vi "BLED1112-Rx Packet parser (EVENT-Connection status).vi"(5 "message package":u8[](array[numeric])=[128, 16, 3, 0, 0, 9, 198, 109, 145, 234, 23, 0, 0, 6, 0, 100, 0, 0, 0, 255] format="%02x") -> (0 "message out":u8[](array[numeric])=[128, 16, 3, 0, 0, 9, 198, 109, 145, 234, 23, 0, 0, 6, 0, 100, 0, 0, 0, 255] format="%02x", 1 "Packet OK":bool, 2 "Data Structure":T1={"Message Type (Response)"=128, "Payload length"=16, "Command Class (System)"=3, "Message ID"=0, "Connection handle"=0, "flags"=9, "Bluetooth address"=[198, 109, 145, 234, 23, 0], "address type"=0, "conn_interval(ms)"=7.5, "timeout(ms)"=1000.0, "latency"=0, "bonding(0xFF)"=255} {"address type" format="%02x" items=["Public", "Random"]; "flags" format="%02x"; "bonding(0xFF)" format="%02x"; "latency" format="%04x"; "Bluetooth address" format="%02x"; "Connection handle" format="%02x"; "Message ID" format="%02x"; "Message Type (Response)" format="%02x" items=["Command / Response"=0, "Event"=128]; "Command Class (System)" format="%02x" items=["System", "Persistent Store", "Attribute database", "Connection", "Attribute client", "Security Manager", "Generic Access Profile", "Hardware"]})   [LabVIEW 2015]
uses:
  Lib_Bled112 toolkit/type_def/message_type.ctl
  Lib_Bled112 toolkit/type_def/message_class.ctl
panel:
  # "Rx Packet parser (EVENT-Connection status)"
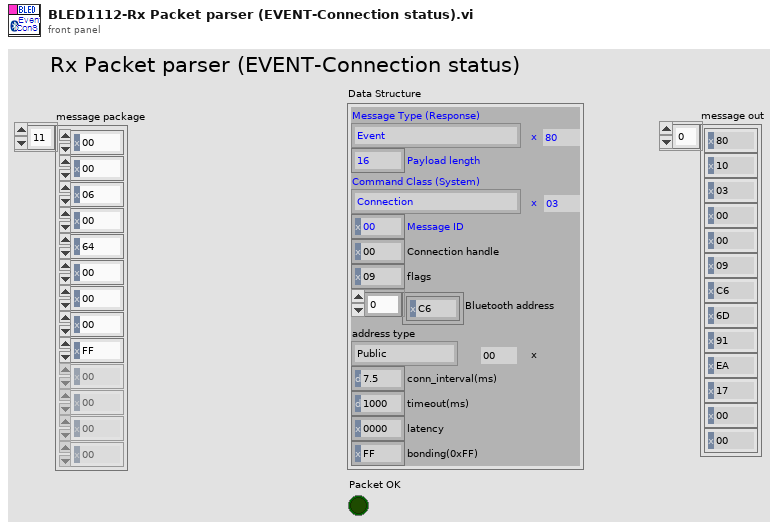
[diagram p1: front panel]
types:
  T1 = typedef "컨트롤-BLED Rx (EVENT-Connection status).ctl" = cluster{"Message Type (Response)":T2, "Payload length":u8, "Command Class (System)":T3, "Message ID":u8, "Connection handle":u8, "flags":u8, "Bluetooth address":u8[], "address type":T3, "conn_interval(ms)":dbl, "timeout(ms)":dbl, "latency":u16, "bonding(0xFF)":u8}
  T2 = typedef "message_type.ctl" = u8
  T3 = typedef "message_class.ctl" = u8
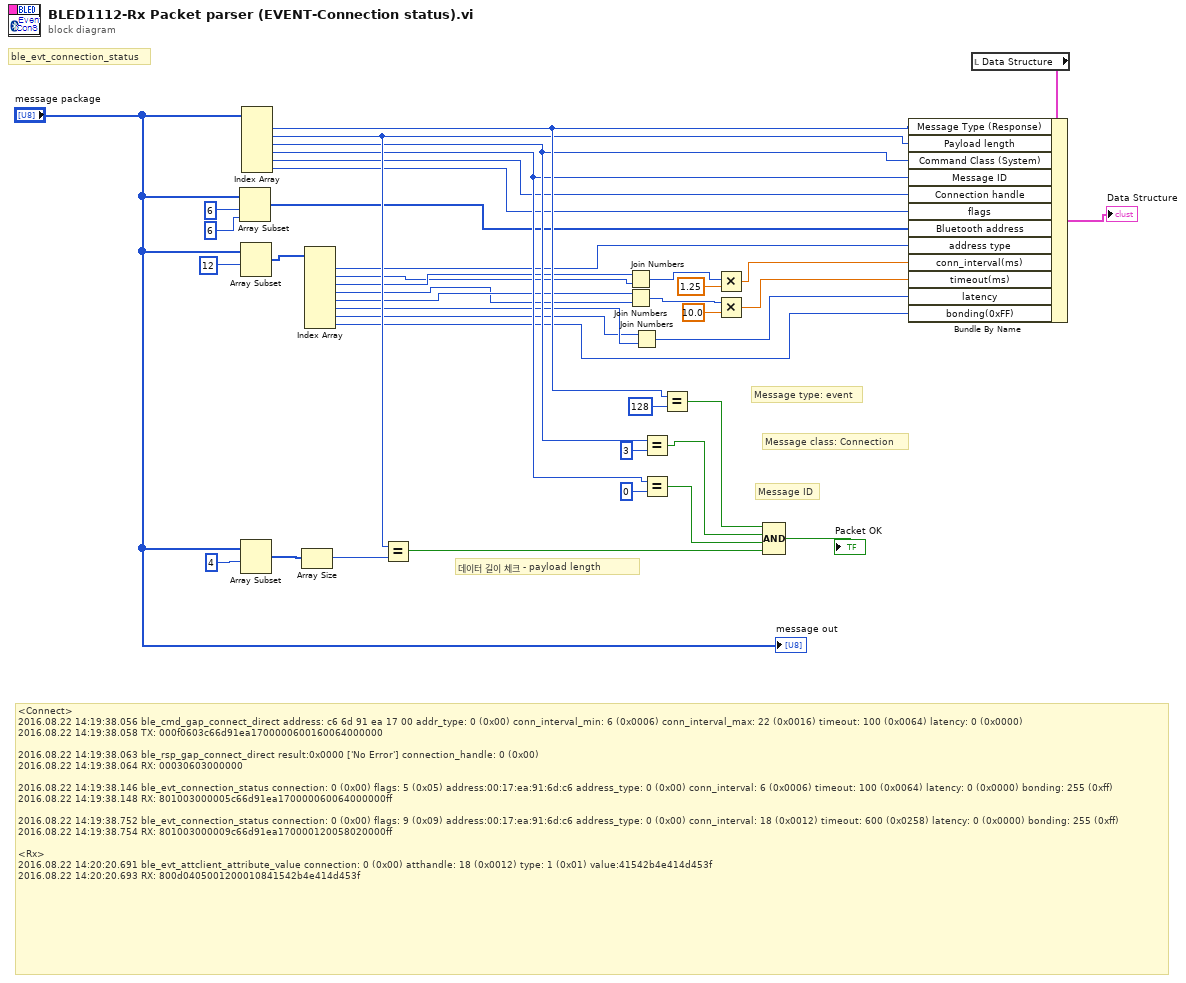
[diagram p0: block diagram]
diagram:
  # "Message type: event"
  # "ble_evt_connection_status"
  # "Message ID"
  # "Message class: Connection"
  # "데이터 길이 체크 - payload length"
  # "<Connect>\n2016.08.22 14:19:38.056 ble_cmd_gap_connect_direct address: c6 6d 91 ea 17 00 addr_type: 0 (0x00) conn_interval_min: 6 (0x0006) conn_interval_max: 22 (0x0016) timeout: 100 (0x0064) latency: 0 (0x0000)\n2016.08.22 14:19:38.058 TX: 000f0603c66d91ea1700000600160064000000\n\n2016.08.22 14:19:38.063 ble_rsp_gap_connect_direct result:0x0000 ['No Error'] connection_handle: 0 (0x00)\n2016.08.22 14:19:38.064 RX: 00030603000000\n\n2016.08.22 14:19:38.146 ble_evt_connection_status connection: 0 (0x00) flags: 5 (0x05) address:00:17:ea:91:6d:c6 address_type: 0 (0x00) conn_interval: 6 (0x0006) timeout: 100 (0x0064) latency: 0 (0x0000) bonding: 255 (0xff)\n2016.08.22 14:19:38.148 RX: 801003000005c66d91ea170000060064000000ff\n\n2016.08.22 14:19:38.752 ble_evt_connection_status connection: 0 (0x00) flags: 9 (0x09) address:00:17:ea:91:6d:c6 address_type: 0 (0x00) conn_interval: 18 (0x0012) timeout: 600 (0x0258) latency: 0 (0x0000) bonding: 255 (0xff)\n2016.08.22 14:19:38.754 RX: 801003000009c66d91ea170000120058020000ff\n\n<Rx>\n2016.08.22 14:20:20.691 ble_evt_attclient_attribute_value connection: 0 (0x00) atthandle: 18 (0x0012) type: 1 (0x01) value:41542b4e414d453f\n2016.08.22 14:20:20.693 RX: 800d0405001200010841542b4e414d453f"
  n1 = Array Subset(array="message package", index=6 ("인덱스"), length=6 ("인덱스")) -> (w12:u8[])
  n2 = Array Subset(array="message package", index=12 ("인덱스")) -> (w31:u8[])  [unwired: 1 in]
  n3 = Array Subset(array="message package", index=4 ("인덱스")) -> (w37:u8[])  [unwired: 1 in]
  n4 = Index Array(array="message package") -> (element #1=w18:u8, element #2=w17:u8, element #3=w16:u8, element #4=w15:u8, element #5=w14:u8, element #6=w13:u8)  [unwired: 6 in]
  n5 = Array Size(array=w37) -> (size(s)=w36:i32)
  n6 = Index Array(array=w31) -> (element #1=w11:u8, element #2=w9:u8, element #3=w10:u8, element #4=w7:u8, element #5=w8:u8, element #6=w4:u8, element #7=w3:u8, element #8=w1:u8)  [unwired: 8 in]
  n7 = Equal?(x=w17, y=w36) -> (x = y?=w39:bool)
  n8 = Join Numbers(hi=w10, lo=w9) -> ((hi.lo)=w25:u16)
  n9 = Join Numbers(hi=w8, lo=w7) -> ((hi.lo)=w23:u16)
  n10 = Join Numbers(hi=w3, lo=w4) -> ((hi.lo)=w2:u16)
  n11 = Equal?(x=w16, y=3 ("인덱스")) -> (x = y?=w27:bool)
  n12 = Equal?(x=w15, y=0 ("인덱스")) -> (x = y?=w28:bool)
  n13 = Equal?(x=w18, y=128 ("인덱스")) -> (x = y?=w21:bool)
  n14 = Multiply(x=w25, y=1.25) -> (x*y=w6:dbl)
  n15 = Multiply(x=w23, y=10.0) -> (x*y=w5:dbl)
  n16 = Compound Arithmetic op=AND ("복합 연산")(w21, w27, w28, w39) -> (→"Packet OK":bool)
  n17 = local read "Data Structure"() -> (w20:T1)
  n18 = Bundle By Name(cluster=w20, "Message Type (Response)"=w18, "Payload length"=w17, "Command Class (System)"=w16, "Message ID"=w15, "Connection handle"=w14, "flags"=w13, "Bluetooth address"=w12, "address type"=w11, "conn_interval(ms)"=w6, "timeout(ms)"=w5, "latency"=w2, "bonding(0xFF)"=w1) -> (→"Data Structure":T1)
  "message out" <- "message package"
